vi "Main HMI.vi"() -> ()   [LabVIEW 2019]
uses:
  Control/State - Main HMI.ctl
  Control/Button Strip.ctl
  Control/Data Struct - Display Data.ctl
  Control/Data Struct - SB.ctl
  Control/Data Struct - Bank.ctl
  Control/Data Struct - SI.ctl
  Control/Data Struct - PM.ctl
  Control/Data Struct - Modbus Reply.ctl
  Control/Device Name.ctl
  Control/Config File Selection.ctl
  Control/State - eFGV.ctl
  Control/State - Query Type.ctl
  Control/Data Type - OPC to SQL.ctl
  43804817-17bc-4d55-847e-17a9177b19d7.vi
  4ba1452d-8fb0-41f4-ac78-9eeaebd610db.vi
  <vilib>/Comparison/Equal/Equal Functor/Equal Functor.lvclass
panel:
  in  "EXIT Button":bool
  out "error out":errorcluster
  in  "error in (no error)":errorcluster
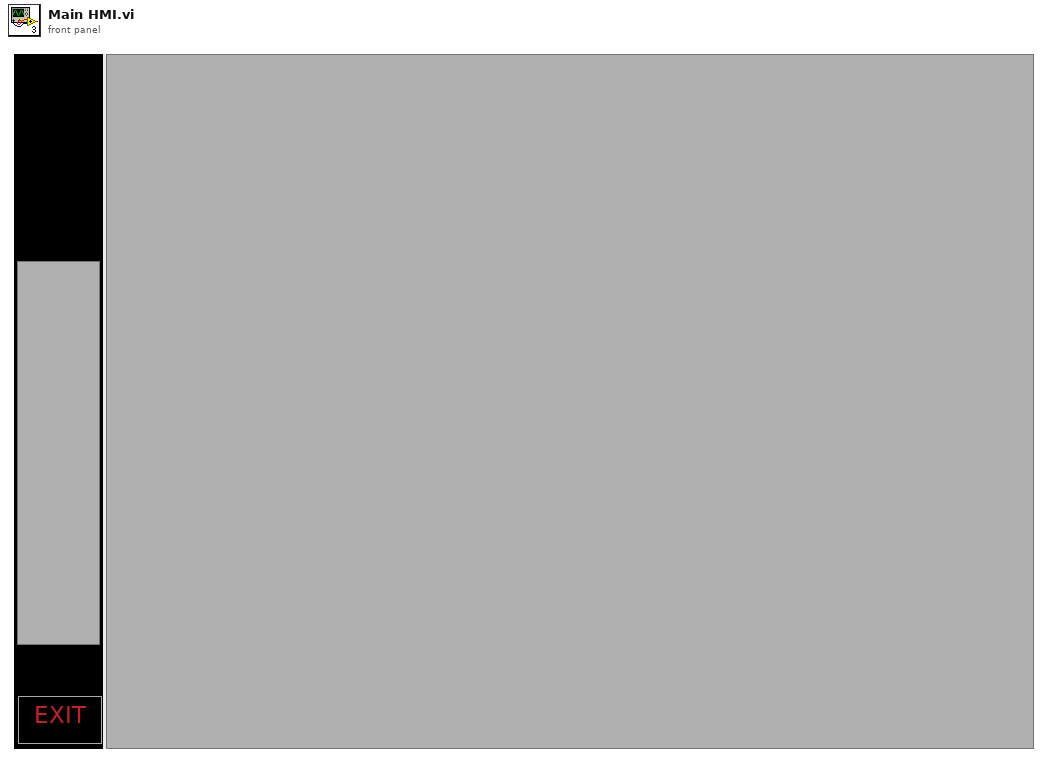
[diagram p1: front panel]
types:
  T1 = typedef "Button Strip.ctl" = enum32{"Home", "Setting", "Alert", "Save", "Chart"}
  T2 = typedef "Data Struct - Display Data.ctl" = cluster{"SB-01":T3, "SB-02":T3, "Bank-01":T4, "Bank-02":T4, "SI-M":T5, "SI-01":T5, "PM-01":T6}
  T3 = typedef "Data Struct - SB.ctl" = cluster{"Pac":dbl, "A.Vdc":dbl, "A.Idc":dbl, "B.Vdc":dbl, "B.Idc":dbl}
  T4 = typedef "Data Struct - Bank.ctl" = cluster{"SOC":dbl, "V_Bat":dbl, "I_Bat":dbl, "T_Bat":dbl}
  T5 = typedef "Data Struct - SI.ctl" = cluster{"Pac":dbl, "L1":dbl, "L2":dbl, "L3":dbl, "Freq":dbl}
  T6 = typedef "Data Struct - PM.ctl" = cluster{"Pac":dbl, "Vac":dbl, "Iac":dbl, "Freq":dbl}
  T7 = typedef "Data Struct - Modbus Reply.ctl" = cluster{"Modbus Req":T8, "Data Output":cluster{"Control Name":string, "Value":dbl}[]}
  T8 = typedef "Device Name.ctl" = enum16{"SB-01", "SB-02", "SB-03", "SB-04", "STP-01", "STP-02", "STP-03", "STP-04", "BANK-01", "BANK-02", "BANK-03", "BANK-04", "SI-M-01", "SI-M-02", "SI-M-03", "SI-M-04", "PM-01", "PM-02", "PM-03", "PM-04"}
  T9 = cluster{"Timeout":i32, "Radio Buttons":T1, "All Module Ref":refnum<vi>[], "Data Struct - All":T2, "SQL Connected":bool, "Modbus Reply":T7, "Home Page Name":string, "Modbus Req":T8, "Accumulated Data":string[][], "Elapsed Time":dbl, "Devices List":T8[]}
  T10 = typedef "State - Main HMI.ctl" = enum16{"Init module", "Register event", "Init eFGV", "Run Module", "Idle", "Change Page", "Request Data from Modbus", "Process Data", "Update Layout", "Send to SQL Module", "Close All Module", "Unregister event", "Close module"}
  T11 = typedef "Config File Selection.ctl" = enum16{"Modbus", "SQL", "General"}
  T12 = typedef "State - eFGV.ctl" = enum16{"Init", "Read", "Write", "Close"}
  T13 = typedef "Data Type - OPC to SQL.ctl" = cluster{"DB Message":string, "DB Command":string, "Module Name":string}
  T14 = typedef "State - Query Type.ctl" = enum16{"SELECT", "UPDATE", "INSERT INTO", "TRUNCATE TABLE"}
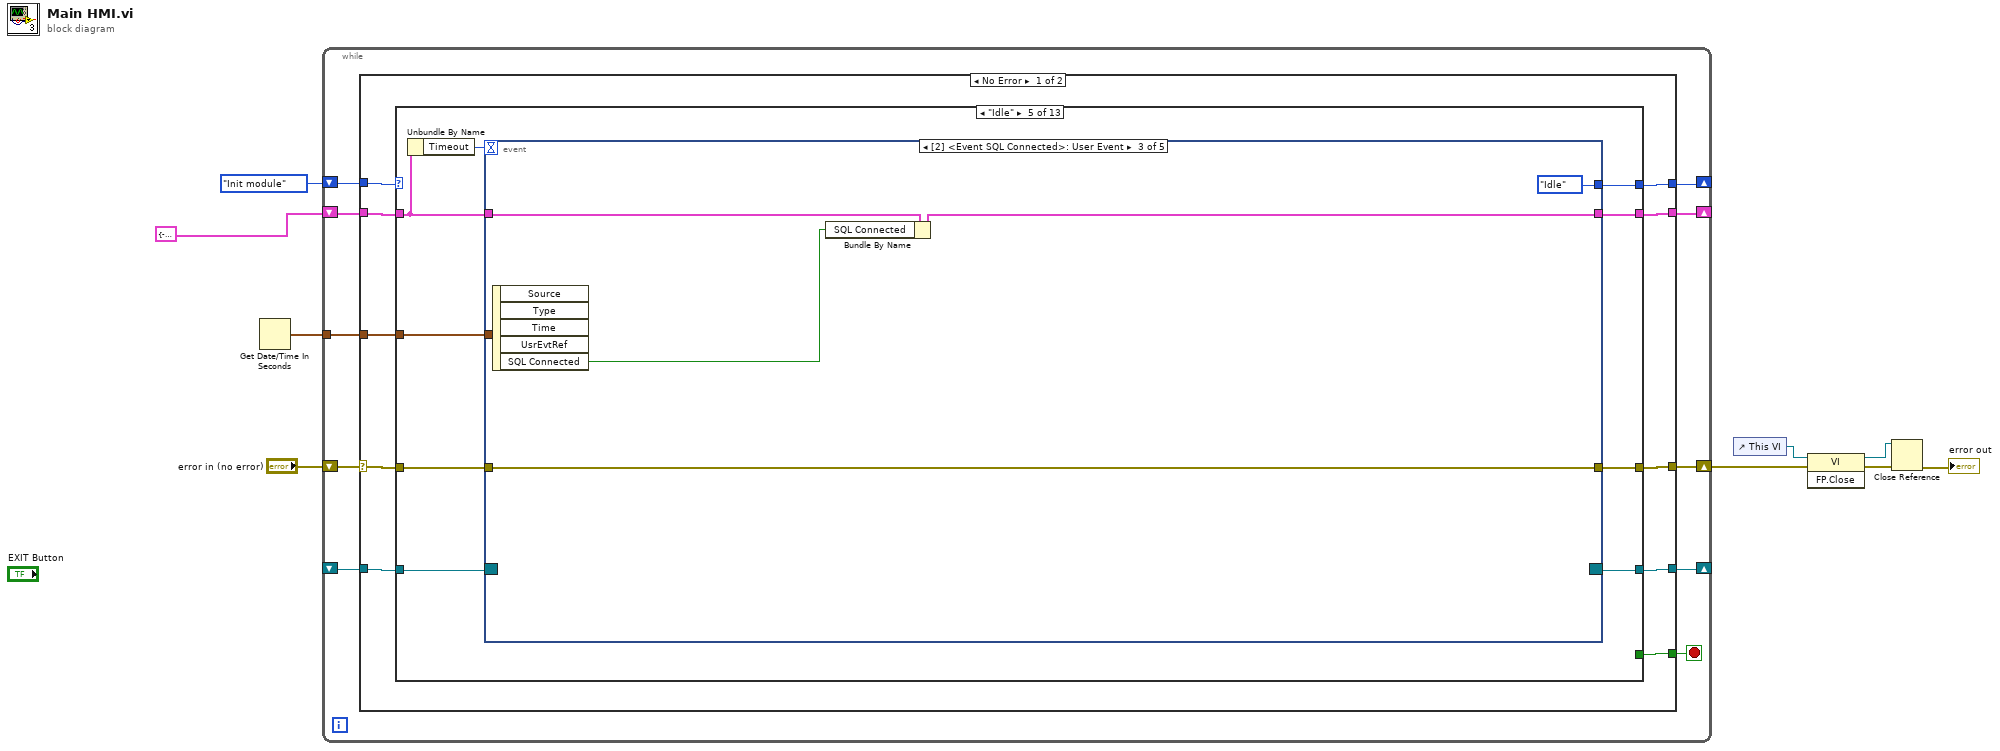
[diagram p0: block diagram]
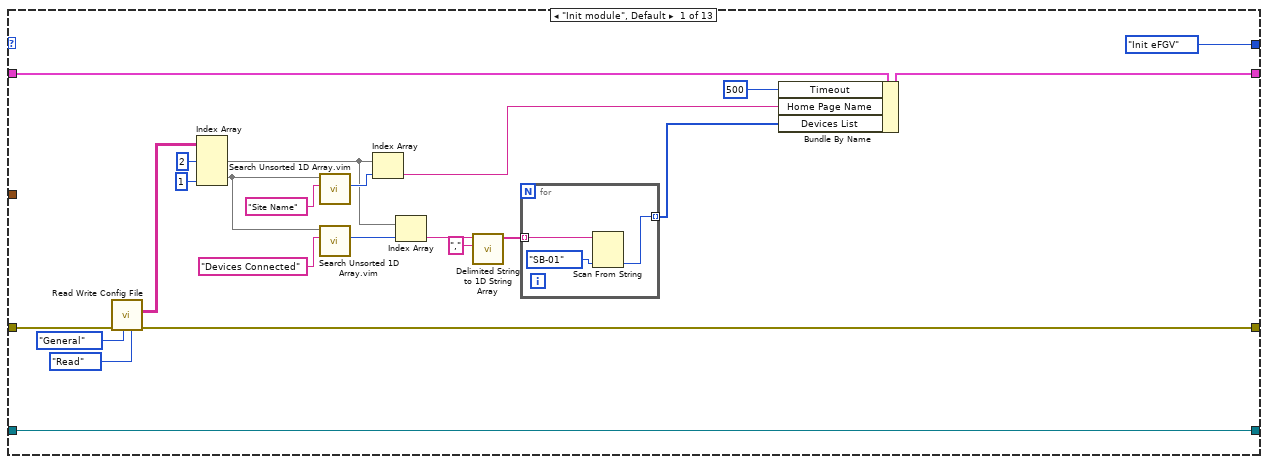
[diagram p2: hidden frame]
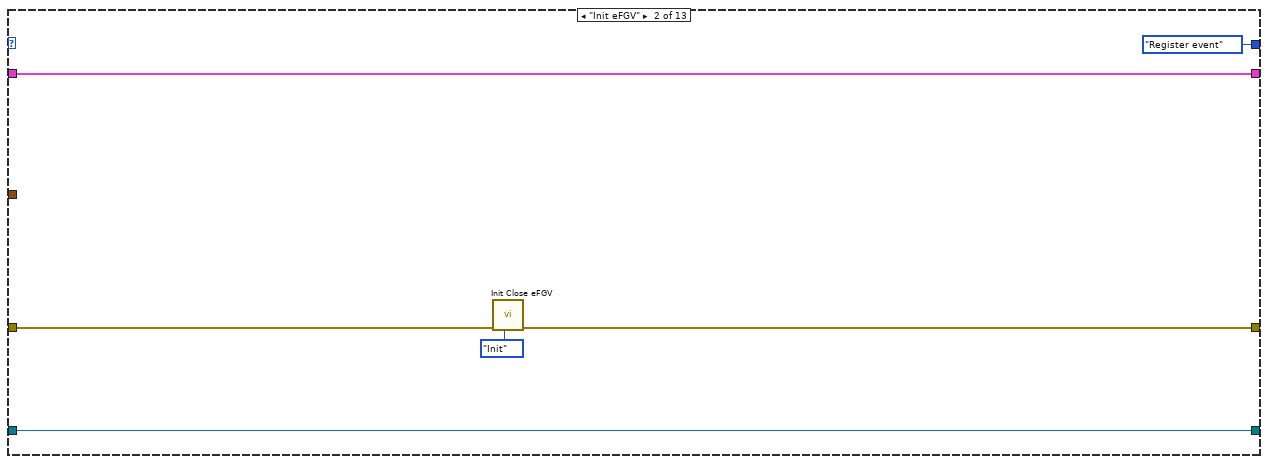
[diagram p3: hidden frame]
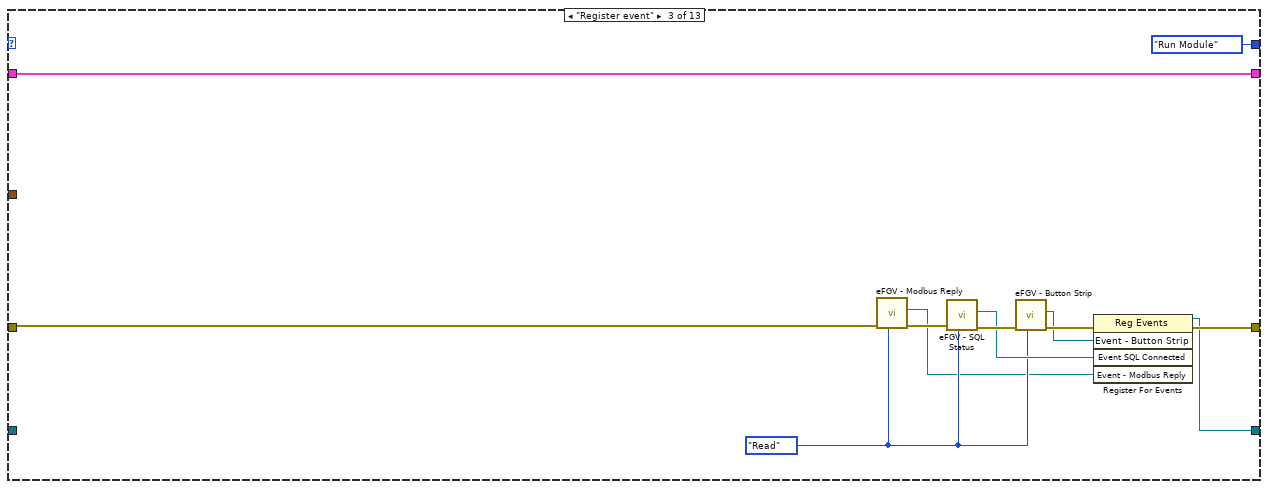
[diagram p4: hidden frame]
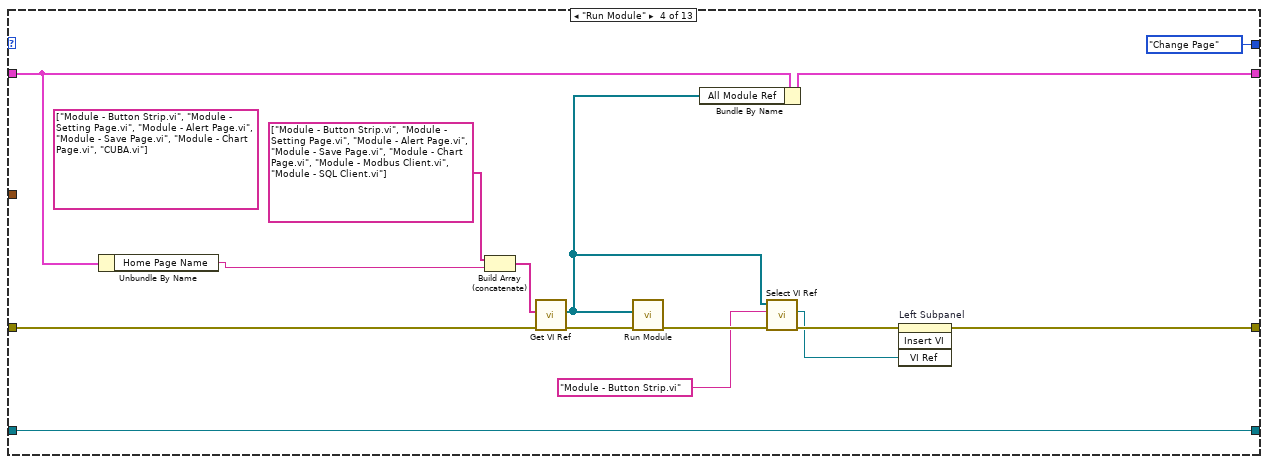
[diagram p5: hidden frame]
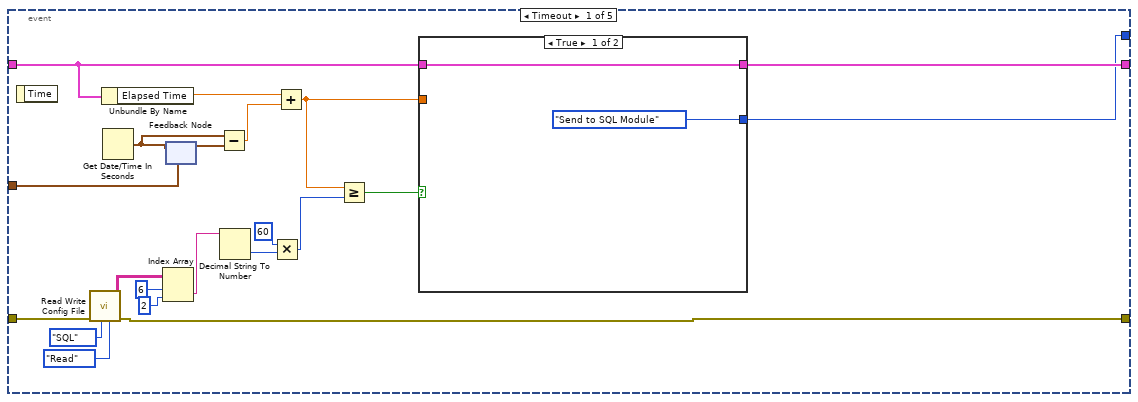
[diagram p6: hidden frame]
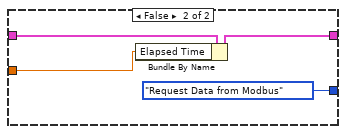
[diagram p7: hidden frame]
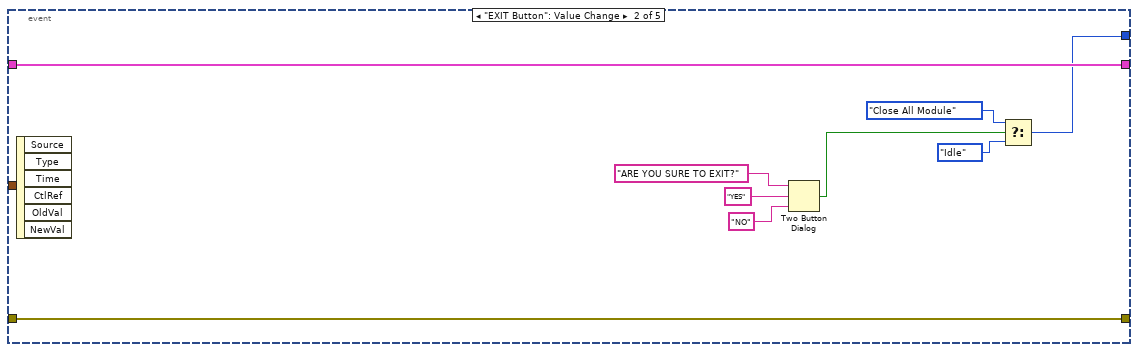
[diagram p8: hidden frame]
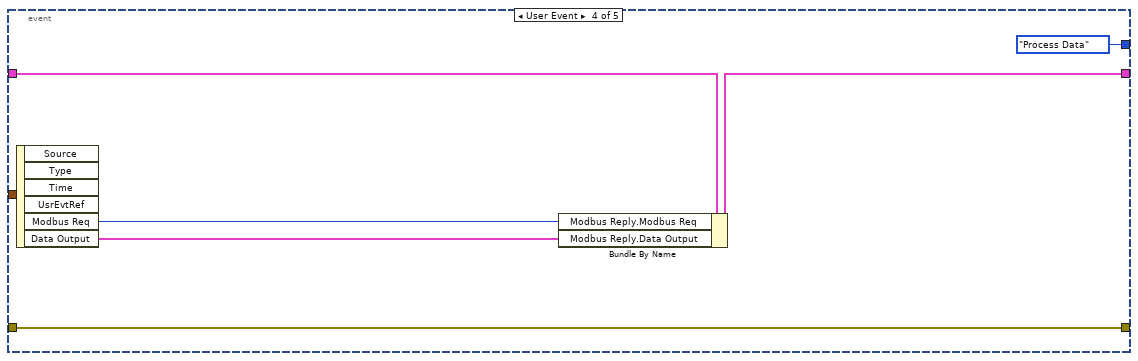
[diagram p9: hidden frame]
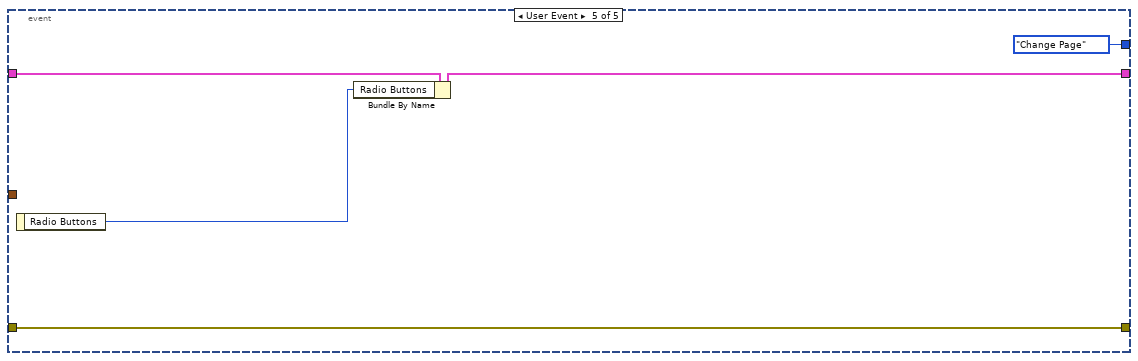
[diagram p10: hidden frame]
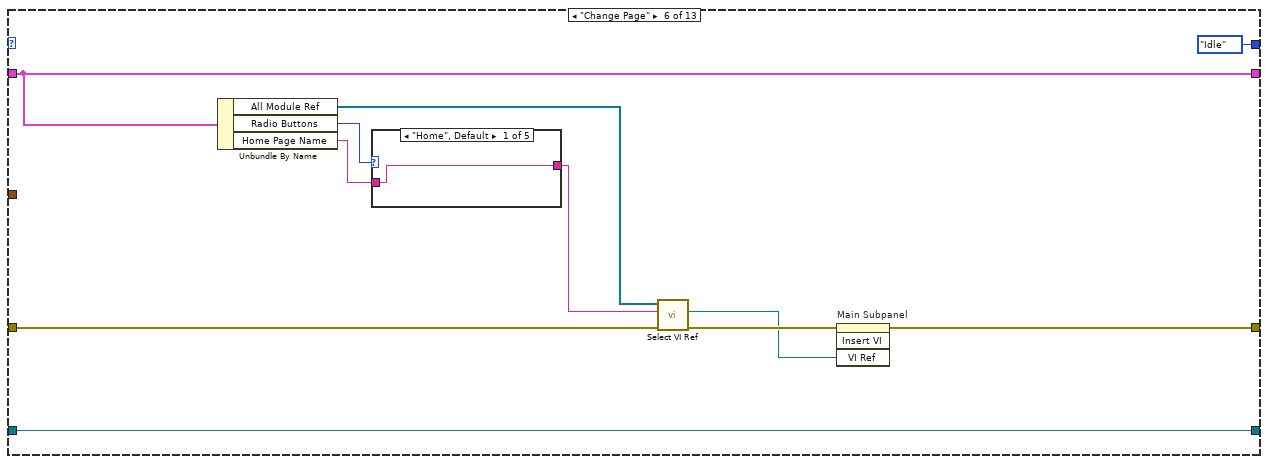
[diagram p11: hidden frame]
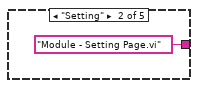
[diagram p12: hidden frame]
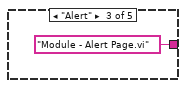
[diagram p13: hidden frame]
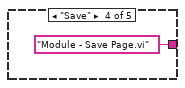
[diagram p14: hidden frame]
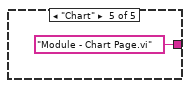
[diagram p15: hidden frame]
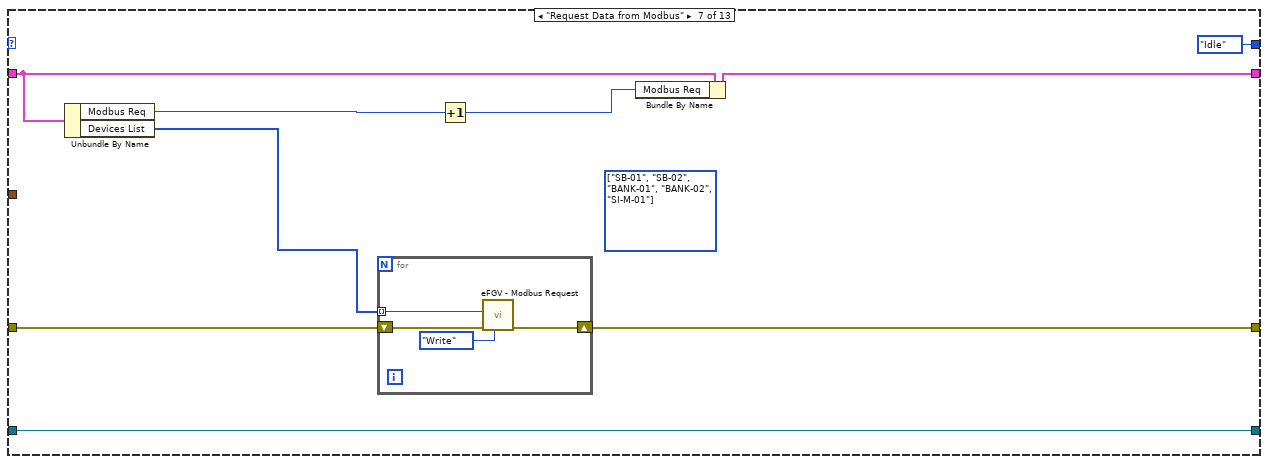
[diagram p16: hidden frame]
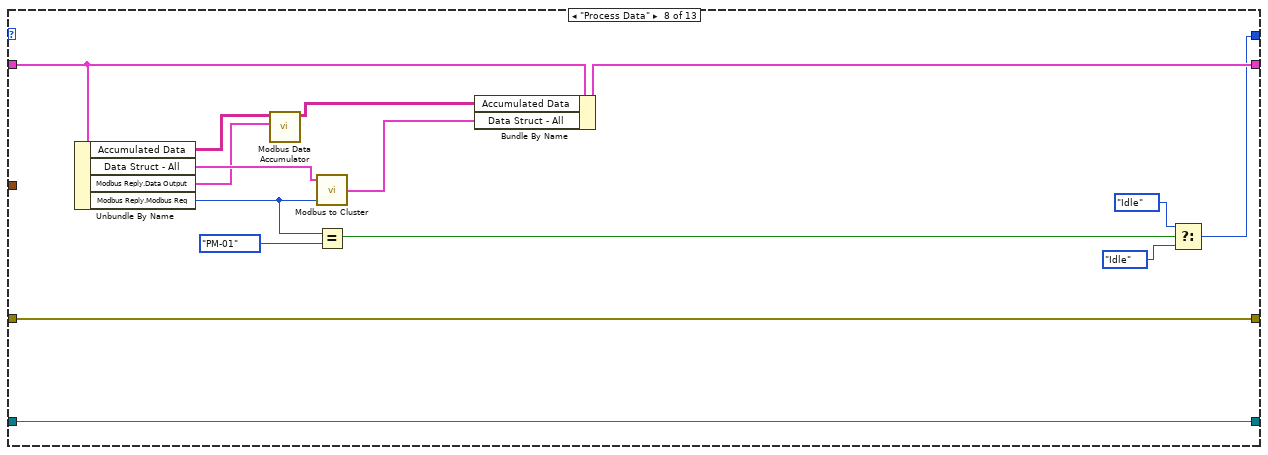
[diagram p17: hidden frame]
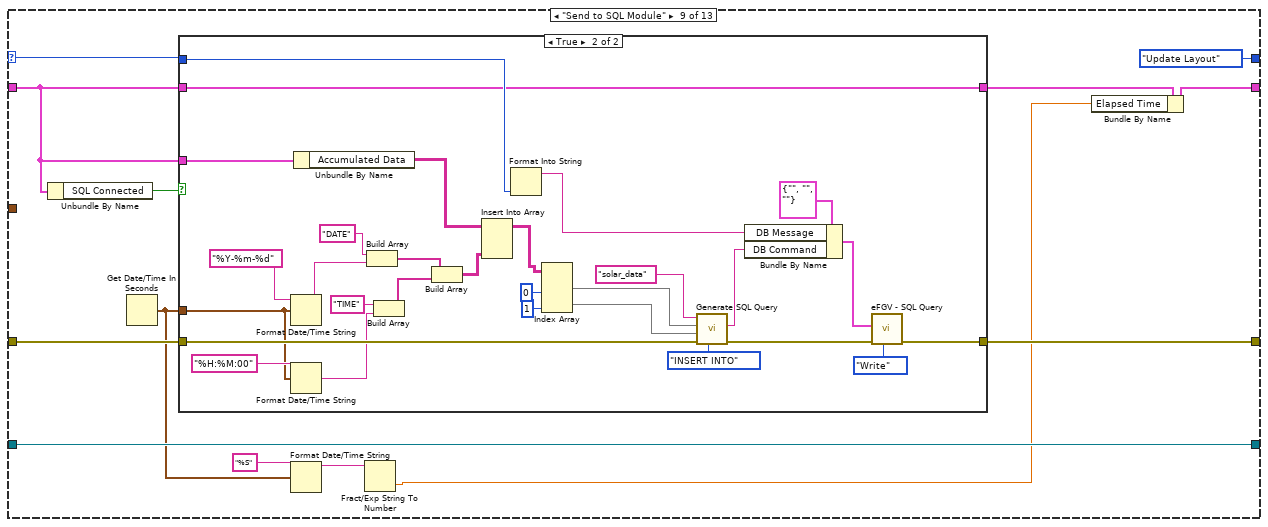
[diagram p18: hidden frame]
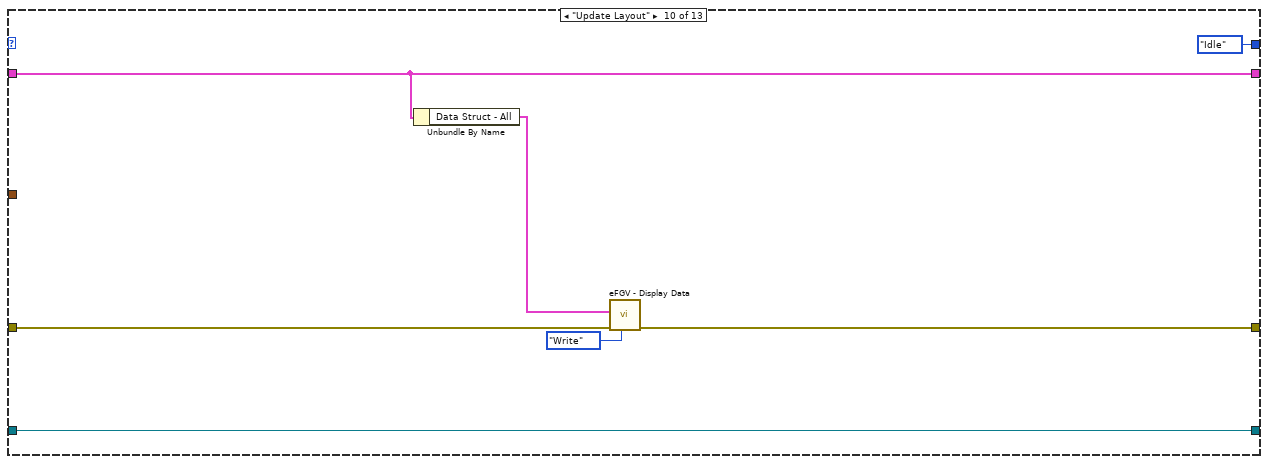
[diagram p20: hidden frame]
diagram:
  n1 = Get Date/Time In Seconds() -> (seconds since 1Jan1904=w6:timestamp)
  n2 = while {
    shift-right: [w17] -> w4
    shift-left: "error in (no error)" -> [w19]
    shift-right: [w13] -> _
    shift-left: State_-_Main_HMI."Init module" -> [w18]
    shift-right: [w15] -> _
    shift-left: T9 {"Timeout"=-1, "Radio Buttons"=enum."Home", "All Module Ref"=[], "Data Struct - All"={"SB-01"={"Pac"=0.0, "A.Vdc"=0.0, "A.Idc"=0.0, "B.Vdc"=0.0, "B.Idc"=0.0}, "SB-02"={"Pac"=0.0, "A.Vdc"=0.0, "A.Idc"=0.0, "B.Vdc"=0.0, "B.Idc"=0.0}, "Bank-01"={"SOC"=0.0, "V_Bat"=0.0, "I_Bat"=0.0, "T_Bat"=0.0}, "Bank-02"={"SOC"=0.0, "V_Bat"=0.0, "I_Bat"=0.0, "T_Bat"=0.0}, "SI-M"={"Pac"=0.0, "L1"=0.0, "L2"=0.0, "L3"=0.0, "Freq"=0.0}, "SI-01"={"Pac"=0.0, "L1"=0.0, "L2"=0.0, "L3"=0.0, "Freq"=0.0}, "PM-01"={"Pac"=0.0, "Vac"=0.0, "Iac"=0.0, "Freq"=0.0}}, "SQL Connected"=FALSE, "Modbus Reply"={"Modbus Req"=enum."SB-01", "Data Output"=[]}, "Home Page Name"="", "Modbus Req"=enum."SB-01", "Accumulated Data"=[], "Elapsed Time"=0.0, "Devices List"=[]} -> [w16]
    shift-right: [w12] -> _
    shift-left: _ -> [w11]
    tunnel: w6 -> [w10]
    stop <- w14 stop-if-true
    n3 = case shown="No Error" w19 {
      selector: w19 -> [w28 w274]
      tunnel: w18 -> [w29 _]
      tunnel: [w27 w270] -> w17
      tunnel: w16 -> [w26 w272]
      tunnel: [w25 w272] -> w15
      tunnel: [w24 _] -> w14
      tunnel: [w23 State_-_Main_HMI."Idle"] -> w13
      tunnel: [w22 w269] -> w12
      tunnel: w11 -> [w21 w269]
      tunnel: w10 -> [w20 _]
      frame No Error {
        n4 = case shown="\"Idle\"" w29 {
          selector: w29 -> [_ _ _ _ _ _ _ _ w202 _ _ _ _]
          tunnel: w28 -> [w47 w58 w64 w87 w94 w157 w172 w179 w204 w241 w252 w262 w268]
          tunnel: [w46 w57 w71 w79 w93 w160 w171 w179 w203 w240 w245 w261 w268] -> w27
          tunnel: w26 -> [w52 w61 w73 w77 w96 w154 w170 w192 w200 w242 w250 w263 w267]
          tunnel: [w50 w61 w73 w85 w95 w154 w169 w190 w195 w242 w250 w263 w267] -> w25
          tunnel: [_ _ _ _ _ _ _ _ _ _ _ _ TRUE] -> w24
          tunnel: [State_-_Main_HMI."Init eFGV" State_-_Main_HMI."Register event" State_-_Main_HMI."Run Module" State_-_Main_HMI."Change Page" w92 State_-_Main_HMI."Idle" State_-_Main_HMI."Idle" w183 State_-_Main_HMI."Update Layout" State_-_Main_HMI."Idle" State_-_Main_HMI."Unregister event" State_-_Main_HMI."Close module" State_-_Main_HMI."Close module"] -> w23
          tunnel: [w48 w59 w70 w86 w90 w159 w173 w193 w205 w243 w251 w259 w264] -> w22
          tunnel: w21 -> [w48 w59 _ w86 w91 w159 w173 w193 w205 w243 w251 w259 w264]
          tunnel: w20 -> [_ _ _ _ w89 _ _ _ _ _ _ _ _]
          frame "Init module", Default {
            n5 = call "Read Write Config File.vi"("Operation"=enum16{"Read", "Write"}."Read", "Config File"=Config_File_Selection."General", "error in (no error)"=w47) -> ("error out"=w46:errorcluster, "Section-Key-Value Out"=w43:string[][])  [unwired: 7 in]
            n6 = Index Array(array=w43, index (col) #1=2 ("disabled index (col)"), index (col) #2=1 ("disabled index (col)")) -> (element #1=w34:string[], element #2=w36:string[])  [unwired: 2 in]
            n7 = call "Search Unsorted 1D Array.vim"("element"="Site Name", "unsorted 1D array"=w36) -> ("index of element"=w39:i32)  [unwired: 9 in]
            n8 = call "Search Unsorted 1D Array.vim"("element"="Devices Connected", "unsorted 1D array"=w36) -> ("index of element"=w35:i32)  [unwired: 9 in]
            n9 = Index Array(array=w34, index=w39) -> (element=w38:string)
            n10 = Index Array(array=w34, index=w35) -> (element=w33:string)
            n11 = call <vilib>:"Delimited String to 1D String Array.vi"("delimiter"=",", "delimited string"=w33) -> ("string array"=w31:string[])  [unwired: 9 in]
            n12 = for {
              tunnel: w31 -> [w55] mode=indexing
              tunnel: [w53] -> w30 mode=indexing
              n13 = Scan From String(input string=w55, default 1=Device_Name."SB-01" ("Modbus Req")) -> (output 1=w53:T8)  [unwired: 3 in, 3 out]
            }
            n14 = Bundle By Name(cluster=w52, "Timeout"=500, "Home Page Name"=w38, "Devices List"=w30) -> (w50:T9)
          }
          frame "Init eFGV" {
            n15 = call "Init Close eFGV.vi"("State - eFGV"=State_-_eFGV."Init", "error in (no error)"=w58) -> ("error out"=w57:errorcluster)  [unwired: 9 in]
          }
          frame "Register event" {
            w63 = State_-_eFGV."Read" ("State - eFGV")
            n16 = call "eFGV - Modbus Reply.vi"("State - eFGV"=w63, "error in (no error)"=w64) -> ("error out"=w65:errorcluster, "Event - Modbus Reply"=w62:refnum<user-event>)  [unwired: 8 in]
            n17 = call "eFGV - SQL Status.vi"("State"=w63, "error in (no error)"=w65) -> ("error out"=w67:errorcluster, "Event SQL Connected"=w66:refnum<user-event>)  [unwired: 8 in]
            n18 = call "eFGV - Button Strip.vi"("State - eFGV"=w63, "error in (no error)"=w67) -> ("error out"=w69:errorcluster, "Event - Button Strip"=w68:refnum<user-event>)  [unwired: 8 in]
            n19 = register-events(error in=w69, w68, w66, w62) -> (reference out=w70:refnum<event-registration>, error out=w71:errorcluster)  [unwired: 1 in]
          }
          frame "Run Module" {
            (unwired) string[] ["Module - Button Strip.vi", "Module - Setting Page.vi", "Module - Alert Page.vi", "Module - Save Page.vi", "Module - Chart Page.vi", "CUBA.vi"] ("Module Names")
            n20 = Unbundle By Name(w77) -> ("Home Page Name"=w76:string)
            n21 = Build Array (concatenate)(string[] ["Module - Button Strip.vi", "Module - Setting Page.vi", "Module - Alert Page.vi", "Module - Save Page.vi", "Module - Chart Page.vi", "Module - Modbus Client.vi", "Module - SQL Client.vi"] ("Module Names"), w76) -> (w75:string[])
            n22 = call "Get VI Ref.vi"("error in (no error)"=w87, "Module Names"=w75) -> ("error out"=w84:errorcluster, "All Module Ref"=w82:refnum<vi>[])  [unwired: 8 in]
            n23 = call "Run Module.vi"("error in (no error)"=w84, "All Module Ref"=w82) -> ("error out"=w83:errorcluster)  [unwired: 9 in]
            n24 = Bundle By Name(cluster=w77, "All Module Ref"=w82) -> (w85:T9)
            n25 = call "Select VI Ref.vi"("error in (no error)"=w83, "Module Name"="Module - Button Strip.vi", "All Module Ref"=w82) -> ("error out"=w80:errorcluster, "VI Refnum"=w78:refnum<vi>)  [unwired: 7 in]
            n26 = invoke on="Left Subpanel" class="SubPnl" method="Insert VI"(error in=w80, "VI Ref"=w78) -> (error out=w79:errorcluster)  [unwired: 2 in, 3 out]
          }
          frame "Idle" {
            n27 = Unbundle By Name(w96) -> ("Timeout"=w97:i32)
            n28 = event shown="[2] <Event SQL Connected>: User Event" {
              selector: w91 -> [_ _ _ _ _]
              dyn-events: [_ _ _ _ _] -> w90
              timeout: w97 -> [_ _ _ _ _]
              tunnel: w96 -> [w102 w129 w138 w139 w149]
              tunnel: [w101 w129 w135 w142 w146] -> w95
              tunnel: w94 -> [w109 w130 w136 w143 w147]
              tunnel: [w108 w130 w136 w143 w147] -> w93
              tunnel: [w100 w126 State_-_Main_HMI."Idle" State_-_Main_HMI."Process Data" State_-_Main_HMI."Change Page"] -> w92
              tunnel: w89 -> [w98 _ _ _ _]
              event Timeout {
                n29 = event-data() -> ()  [unwired: 1 in, 1 out]
                n30 = call "Read Write Config File.vi"("Operation"=enum16{"Read", "Write"}."Read", "Config File"=Config_File_Selection."SQL", "error in (no error)"=w109) -> ("error out"=w108:errorcluster, "Section-Key-Value Out"=w112:string[][])  [unwired: 7 in]
                n31 = Unbundle By Name(w102) -> ("Elapsed Time"=w116:dbl)
                n32 = Get Date/Time In Seconds() -> (seconds since 1Jan1904=w118:timestamp)
                n33 = Index Array(array=w112, index (row)=6 ("disabled index (row)"), index (col)=2 ("disabled index (col)")) -> (element=w107:string)
                n34 = feedback #1(w98) -> (w117:timestamp)
                n35 = feedback-in #1(w118) -> ()
                n36 = Subtract(x=w118, y=w117) -> (x-y=w115:dbl)
                n37 = Decimal String To Number(string=w107) -> (number=w106:i32)  [unwired: 2 in, 1 out]
                n38 = Multiply(x=60, y=w106) -> (x*y=w104:i32)
                n39 = Add(x=w116, y=w115) -> (x+y=w99:dbl)
                n40 = Greater Or Equal?(x=w99, y=w104) -> (x >= y?=w103:bool)
                n41 = case shown="True" w103 {
                  tunnel: w102 -> [w120 w124]
                  tunnel: [w120 w122] -> w101
                  tunnel: [State_-_Main_HMI."Send to SQL Module" State_-_Main_HMI."Request Data from Modbus"] -> w100
                  tunnel: w99 -> [_ w121]
                  frame True {
                  }
                  frame False {
                    n42 = Bundle By Name(cluster=w124, "Elapsed Time"=w121) -> (w122:T9)
                  }
                }
              }
              event "EXIT Button": Value Change {
                n43 = event-data() -> ()  [unwired: 1 in, 6 out]
                n44 = Two Button Dialog(message="ARE YOU SURE TO EXIT?", 1:"NO" ("F button name (\"Cancel\")"), 2:"YES" ("T button name (\"OK\")")) -> (T button?=w125:bool)
                n45 = Select(t=State_-_Main_HMI."Close All Module", s=w125, f=State_-_Main_HMI."Idle") -> (s? t:f=w126:T10)
              }
              event User Event {
                n46 = event-data() -> ("SQL Connected"=w134:bool)  [unwired: 1 in, 4 out]
                n47 = Bundle By Name(cluster=w138, "SQL Connected"=w134) -> (w135:T9)
              }
              event User Event {
                n48 = event-data() -> ("Modbus Req"=w141:T8, "Data Output"=w140:cluster{"Control Name":string, "Value":dbl}[])  [unwired: 1 in, 4 out]
                n49 = Bundle By Name(cluster=w139, "Modbus Reply.Modbus Req"=w141, "Modbus Reply.Data Output"=w140) -> (w142:T9)
              }
              event User Event {
                n50 = event-data() -> ("Radio Buttons"=w145:T1)  [unwired: 1 in]
                n51 = Bundle By Name(cluster=w149, "Radio Buttons"=w145) -> (w146:T9)
              }
            }
          }
          frame "Change Page" {
            n52 = Unbundle By Name(w154) -> ("All Module Ref"=w153:refnum<vi>[], "Radio Buttons"=w152:T1, "Home Page Name"=w150:string)
            n53 = case shown="\"Home\", Default" w152 {
              tunnel: [w161 "Module - Setting Page.vi" "Module - Alert Page.vi" "Module - Save Page.vi" "Module - Chart Page.vi"] -> w151
              tunnel: w150 -> [w161 _ _ _ _]
              frame "Home", Default {
              }
              frame "Setting" {
              }
              frame "Alert" {
              }
              frame "Save" {
              }
              frame "Chart" {
              }
            }
            n54 = call "Select VI Ref.vi"("error in (no error)"=w157, "Module Name"=w151, "All Module Ref"=w153) -> ("error out"=w156:errorcluster, "VI Refnum"=w155:refnum<vi>)  [unwired: 7 in]
            n55 = invoke on="Main Subpanel" class="SubPnl" method="Insert VI"(error in=w156, "VI Ref"=w155) -> (error out=w160:errorcluster)  [unwired: 2 in, 3 out]
          }
          frame "Request Data from Modbus" {
            (unwired) T8[] [enum."SB-01", enum."SB-02", enum."BANK-01", enum."BANK-02", enum."SI-M-01"] items=["SB-01", "SB-02", "SB-03", "SB-04", "STP-01", "STP-02", "STP-03", "STP-04", "BANK-01", "BANK-02", "BANK-03", "BANK-04", "SI-M-01", "SI-M-02", "SI-M-03", "SI-M-04", "PM-01", "PM-02", "PM-03", "PM-04"]
            n56 = Unbundle By Name(w170) -> ("Modbus Req"=w168:T8, "Devices List"=w166:T8[])
            n57 = for {
              tunnel: w166 -> [w175] mode=indexing
              shift-right: [w177] -> w171
              shift-left: w172 -> [w178]
              n58 = call "eFGV - Modbus Request.vi"("State - eFGV"=State_-_eFGV."Write", "error in (no error)"=w178, "Modbus Req"=w175) -> ("error out"=w177:errorcluster)  [unwired: 7 in, 1 out]
            }
            n59 = Increment(x=w168) -> (x+1=w167:T8)
            n60 = Bundle By Name(cluster=w170, "Modbus Req"=w167) -> (w169:T9)
          }
          frame "Process Data" {
            n61 = Unbundle By Name(w192) -> ("Accumulated Data"=w182:string[][], "Data Struct - All"=w191:T2, "Modbus Reply.Data Output"=w181:cluster{"Control Name":string, "Value":dbl}[], "Modbus Reply.Modbus Req"=w188:T8)
            n62 = call "Modbus Data Accumulator.vi"("Modbus Data"=w181, "Accumulated Data"=w182) -> ("Accumulated Data Out"=w180:string[][])  [unwired: 9 in]
            n63 = call "Modbus to Cluster.vi"("Modbus Req"=w188, "Data Struct - All"=w191) -> ("Data Struct - All Out"=w189:T2)  [unwired: 1 in]
            n64 = Equal?(x=w188, y=Device_Name."PM-01") -> (x = y?=w186:bool)
            n65 = Bundle By Name(cluster=w192, "Accumulated Data"=w180, "Data Struct - All"=w189) -> (w190:T9)
            n66 = Select(t=State_-_Main_HMI."Idle", s=w186, f=State_-_Main_HMI."Idle") -> (s? t:f=w183:T10)
          }
          frame "Send to SQL Module" {
            n67 = Unbundle By Name(w200) -> ("SQL Connected"=w201:bool)
            n68 = Get Date/Time In Seconds() -> (seconds since 1Jan1904=w197:timestamp)
            n69 = case shown="True" w201 {
              tunnel: w204 -> [w208 w235]
              tunnel: [w208 w233] -> w203
              tunnel: w202 -> [_ w229]
              tunnel: w200 -> [_ w226]
              tunnel: w200 -> [w207 w210]
              tunnel: [w207 w210] -> w199
              tunnel: w197 -> [_ w209]
              frame False {
              }
              frame True {
                n70 = Format Date/Time String(time format string (%c)="%Y-%m-%d", seconds (now)=w209) -> (date/time string=w217:string)  [unwired: 1 in]
                n71 = Format Date/Time String(time format string (%c)="%H:%M:00", seconds (now)=w209) -> (date/time string=w215:string)  [unwired: 1 in]
                n72 = Unbundle By Name(w226) -> ("Accumulated Data"=w221:string[][])
                n73 = Build Array("DATE", w217) -> (w213:string[])
                n74 = Build Array("TIME" ("element"), w215) -> (w212:string[])
                n75 = Build Array(w213, w212) -> (w211:string[][])
                n76 = Insert Into Array(array=w221, new element=w211) -> (w220:string[][])  [unwired: 2 in]
                n77 = Format Into String(w229) -> (resulting string=w228:string)  [unwired: 3 in, 1 out]
                n78 = Index Array(array=w220, index (col) #1=0 ("disabled index (col)"), index (col) #2=1 ("index (col)")) -> (element #1=w223:string[], element #2=w222:string[])  [unwired: 2 in]
                n79 = call "Generate SQL Query.vi"("Query type"=State_-_Query_Type."INSERT INTO", "error in (no error)"=w235, "Values"=w222, "Column Name"=w223, "Table Name"="solar_data") -> ("error out"=w234:errorcluster, "Query String"=w231:string)  [unwired: 5 in]
                n80 = Bundle By Name(cluster=T13 {"DB Message"="", "DB Command"="", "Module Name"=""} ("OPC to SQL"), "DB Message"=w228, "DB Command"=w231) -> (w230:T13)
                n81 = call "eFGV - SQL Query.vi"("State"=State_-_eFGV."Write", "error in (no error)"=w234, "OPC to SQL"=w230) -> ("error out"=w233:errorcluster)  [unwired: 7 in, 1 out]
              }
            }
            n82 = Format Date/Time String(time format string (%c)="%S", seconds (now)=w197) -> (date/time string=w196:string)  [unwired: 1 in]
            n83 = Fract/Exp String To Number(string=w196) -> (number=w194:dbl)  [unwired: 3 in, 1 out]
            n84 = Bundle By Name(cluster=w199, "Elapsed Time"=w194) -> (w195:T9)
          }
          frame "Update Layout" {
            n85 = Unbundle By Name(w242) -> ("Data Struct - All"=w238:T2)
            n86 = call "eFGV - Display Data.vi"("State - eFGV"=State_-_eFGV."Write", "error in (no error)"=w241, "Display Data"=w238) -> ("error out"=w240:errorcluster)  [unwired: 7 in, 1 out]
          }
          frame "Close All Module" {
            n87 = flat-sequence {
              tunnel: w252 -> [w258]
              tunnel: [w255] -> w249
              frame #0 {
                n88 = call "eFGV - Stop Program.vi"("State - eFGV"=State_-_eFGV."Write", "error in (no error)"=w258, "Stop Program"=TRUE) -> ("error out"=w255:errorcluster)  [unwired: 7 in, 1 out]
                n89 = Wait (ms)(milliseconds to wait=u32 2000) -> ()  [unwired: 1 out]
              }
            }
            n90 = Unbundle By Name(w250) -> ("All Module Ref"=w248:refnum<vi>[])
            n91 = Close Reference(reference=w248, error in (no error)=w249) -> (error out=w246:errorcluster)
            n92 = call "Init Close eFGV.vi"("State - eFGV"=State_-_eFGV."Close", "error in (no error)"=w246) -> ("error out"=w245:errorcluster)  [unwired: 9 in]
          }
          frame "Unregister event" {
            n93 = Unregister For Events(event registration refnum=w259, error in=w262) -> (error out=w261:errorcluster)
          }
          frame "Close module" {
          }
        }
      }
      frame Error {
        n94 = call <vilib>:"Simple Error Handler.vi"("error in (no error)"=w274) -> ("error out"=w273:errorcluster)  [unwired: 4 in, 4 out]
        n95 = call <vilib>:"Clear Errors.vi"("error in (no error)"=w273) -> ("error out"=w270:errorcluster)  [unwired: 5 in, 1 out]
      }
    }
  }
  n96 = control-ref of="This VI"() -> (w5:refnum<vi>)
  n97 = invoke class="VI" method="FP.Close"(reference=w5, error in=w4) -> (reference out=w1:refnum<vi>, error out=w3:errorcluster)  [unwired: 1 in, 1 out]
  n98 = Close Reference(reference=w1, error in (no error)=w3) -> (error out=→"error out":errorcluster)
